vi "Pre Launch Init.vi"(11 "RootModel in":refnum<class "RootModel.lvclass">) -> (0 "error out":errorcluster, 3 "RootModel out":refnum<class "RootModel.lvclass">)   [LabVIEW 2019, in "RootModel.lvlib" / "RootModel.lvclass"]
uses:
  <vilib>/gpm_packages/@cs/mva-core/Source/RootModel/RootModel/RootModel.lvclass
  C:/Program Files/National Instruments/LabVIEW 2019/vi.lib/ActorFramework/Actor/Actor.lvclass
  <vilib>/gpm_packages/@cs/mva-core/Source/RootModel/RootModel/RootModel.lvclass/RootModel.ctl
  <vilib>/gpm_packages/@cs/mva-core/Source/RootModel/RootModel Messages/Run Headless Msg/Run Headless Msg.lvclass
  C:/Program Files/National Instruments/LabVIEW 2019/vi.lib/ActorFramework/Message/Message.lvclass
  <vilib>/ActorFramework/Actor/Actor.lvclass/Actor.ctl
  <vilib>/ActorFramework/Message Enqueuer/Message Enqueuer.lvclass/Message Enqueuer.ctl
  <vilib>/ActorFramework/Message Enqueuer/Message Priority.ctl
  <vilib>/ActorFramework/Message Enqueuer/Init from Existing Queue.vi
  <vilib>/ActorFramework/Message Priority Queue/Priority Enqueue.vi
  <vilib>/ActorFramework/Message Enqueuer/Message Enqueuer.lvclass
  <vilib>/gpm_packages/@cs/mva-core/Source/IModel/IModel/IModel.lvclass
  <vilib>/ActorFramework/Actor/Actor.lvclass
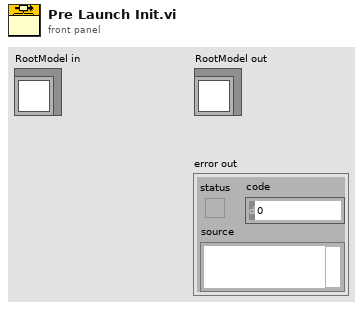
[diagram p1: front panel]
types:
  T1 = typedef "Actor Framework.lvlib/Message Enqueuer.lvclass/Message Priority.ctl" = enum16{"Low", "Normal", "High"}
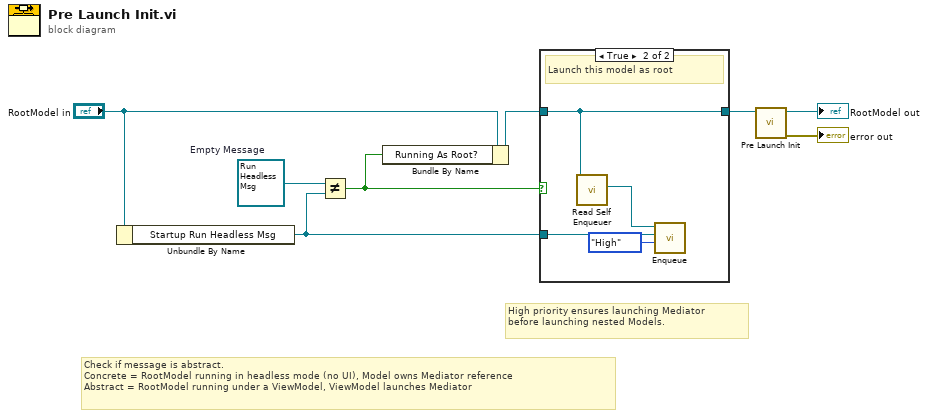
[diagram p0: block diagram]
diagram:
  w7 = refnum<class "Run Headless Msg.lvclass"> refnum  # Empty Message
  # "High priority ensures launching Mediator\nbefore launching nested Models."
  # "Check if message is abstract.\nConcrete = RootModel running in headless mode (no UI), Model owns Mediator reference\nAbstract = RootModel running under a ViewModel, ViewModel launches Mediator"
  n1 = Unbundle By Name("RootModel in") -> ("Startup Run Headless Msg"=w5:refnum<class "Run Headless Msg.lvclass">)
  n2 = Not Equal?(x=w7, y=w5) -> (x != y?=w1:bool)
  n3 = Bundle By Name(cluster="RootModel in", "Running As Root?"=w1) -> (w2:refnum<class "RootModel.lvclass">)
  n4 = case shown="True" w1 {
    tunnel: w5 -> [_ w13]
    tunnel: w2 -> [w9 w10]
    tunnel: [w9 w10] -> w3
    frame False {
      # "NOT running as root"
    }
    frame True {
      # "Launch this model as root"
      n5 = call <vilib>:"Read Self Enqueuer.vi"("Actor"=w10) -> ("Self Enqueuer"=w11:refnum<class "Message Enqueuer.lvclass">)  [unwired: 10 in]
      n6 = call <vilib>:"Enqueue.vi"("Message Priority (Normal)"=Message_Priority."High", "Message"=w13, "Message Enqueuer in"=w11) -> ()  [unwired: 7 in, 2 out]
    }
  }
  n7 = call-parent "Pre Launch Init.vi"("IModel in"=w3) -> ("error out"=→"error out":errorcluster, "IModel out"=→"RootModel out":refnum<class "RootModel.lvclass">)  [unwired: 9 in]
